vi "Actor Core.vi"(8 "error in":errorcluster, 11 "Car Wash Controller in":refnum<class "Vehicle Position Simulation Actor.lvclass">) -> (0 "error out":errorcluster, 3 "Actor out":refnum<class "Actor.lvclass">)   [LabVIEW 2019, in "Vehicle Position Sinmulation Actor.lvlib" / "Vehicle Position Simulation Actor.lvclass"]
doc: "(<B>Filename</B>: Actor Framework.lvlib:Actor.lvclass:Actor Core.vi)\n\nReceives messages to the actor, reacts to them, and initiates any error handling that may shut the actor down.\n\nDescendant classes may override this VI to append parallel tasks for the actor to complete while it handles messages. Overrides use the Call Parent Method node."
uses:
  Vehicle Position Simulation Actor.lvclass
  <vilib>/ActorFramework/Stop Msg/Stop Msg.lvclass
  <vilib>/ActorFramework/Actor/Actor.lvclass
  Vehicle Position Interface/Vehicle Position Interface/Vehicle Position Interface.lvclass
  C:/Workspace/CLA/Carwasher AF 2nd/Vehicle Position Interface/Vehicle Position Interface/Vehicle Position Interface.lvclass
  C:/Program Files (x86)/National Instruments/LabVIEW 2019/vi.lib/ActorFramework/Actor/Actor.lvclass
panel:
  in  "Vehicle Position Simulation":u8(slide) scale=0.0..4.0
  # "UI4"
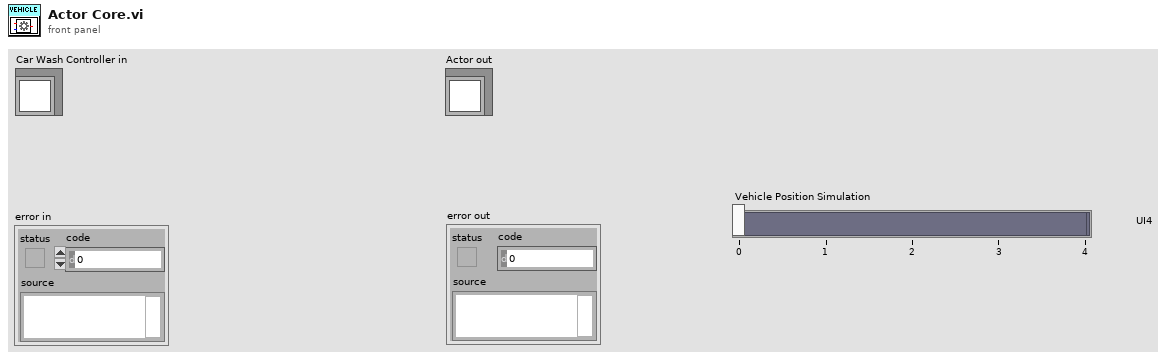
[diagram p1: front panel]
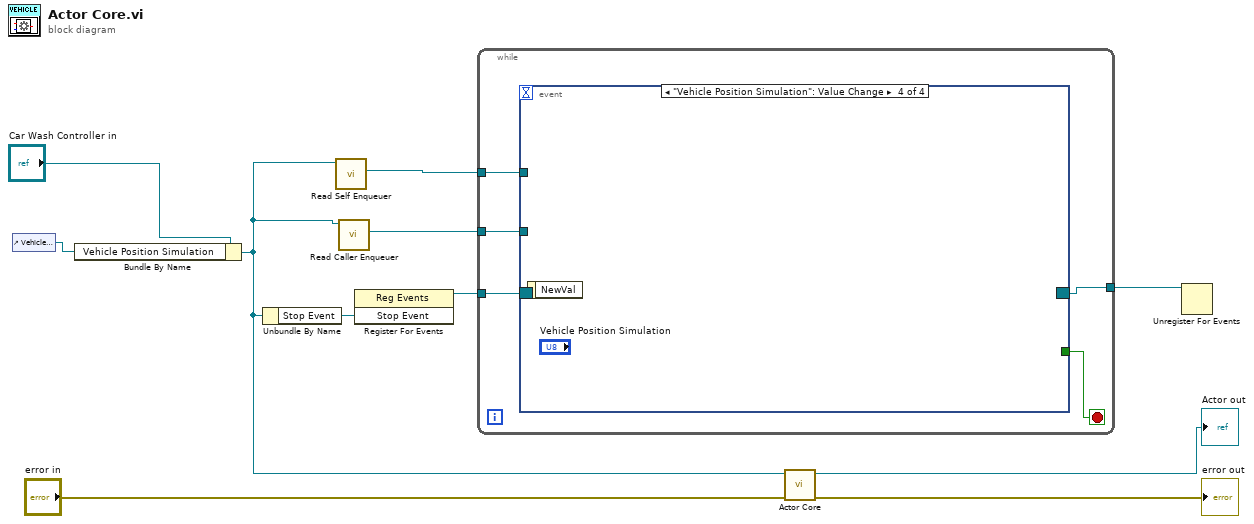
[diagram p0: block diagram]
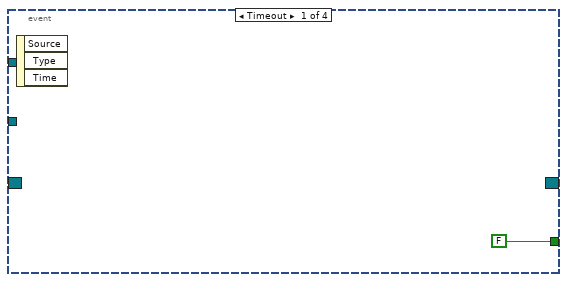
[diagram p2: hidden frame]
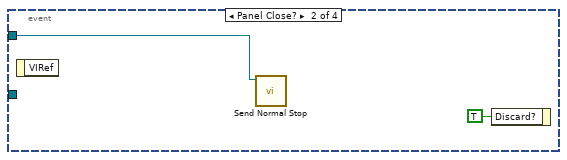
[diagram p3: hidden frame]
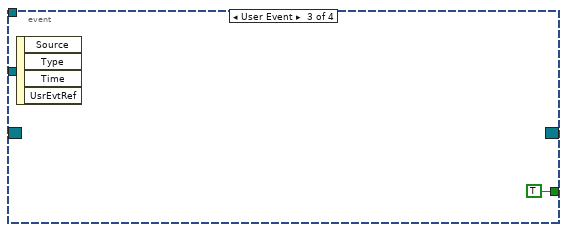
[diagram p4: hidden frame]
diagram:
  n1 = control-ref of="Vehicle Position Simulation"() -> (w3:refnum<vi>)
  n2 = Bundle By Name(cluster="Car Wash Controller in", "Vehicle Position Simulation"=w3) -> (w2:refnum<class "Vehicle Position Simulation Actor.lvclass">)
  n3 = Unbundle By Name(w2) -> ("Stop Event"=w5:refnum<user-event>)
  n4 = call <vilib>:"Read Self Enqueuer.vi"("Actor"=w2) -> ("Self Enqueuer"=w6:refnum<class "Message Enqueuer.lvclass">)  [unwired: 10 in]
  n5 = call <vilib>:"Read Caller Enqueuer.vi"("Actor"=w2) -> ("Caller Enqueuer"=w1:refnum<class "Message Enqueuer.lvclass">)  [unwired: 10 in]
  n6 = register-events(w5) -> (reference out=w8:refnum<event-registration>)  [unwired: 2 in, 1 out]
  n7 = while {
    tunnel: w8 -> [w15]
    tunnel: [w14] -> w7
    tunnel: w6 -> [w13]
    tunnel: w1 -> [w12]
    stop <- w16 stop-if-true
    n8 = event shown="[3] \"Vehicle Position Simulation\": Value Change" {
      selector: w15 -> [_ _ _ _]
      dyn-events: [_ _ _ _] -> w14
      timeout: _ -> [_ _ _ _]
      tunnel: [FALSE _ TRUE _] -> w16
      tunnel: w13 -> [_ w18 _ _]
      tunnel: w12 -> [_ _ _ _]
      event Timeout {
        n9 = event-data() -> ()  [unwired: 1 in, 3 out]
      }
      event Panel Close? {
        n10 = event-data() -> ()  [unwired: 1 in, 1 out]
        n11 = call <vilib>:"Send Normal Stop.vi"("Message Enqueuer"=w18) -> ()  [unwired: 10 in, 1 out]
        n12 = event-data("Discard?"=TRUE) -> ()  [unwired: 1 in, 1 out]
      }
      event User Event {
        n13 = event-data() -> ()  [unwired: 1 in, 4 out]
      }
      event "Vehicle Position Simulation": Value Change {
        n14 = event-data() -> ()  [unwired: 1 in, 1 out]
      }
    }
  }
  n15 = call-parent "Actor Core.vi"("error in"="error in", "Actor in"=w2) -> ("error out"=→"error out":errorcluster, "Actor out"=→"Actor out":refnum<class "Actor.lvclass">)  [unwired: 8 in]
  n16 = Unregister For Events(event registration refnum=w7) -> ()  [unwired: 1 in, 1 out]
